vi "DidMotorCompleteWithoutError.vi"(8 "error in (no error)":errorcluster, 11 "MotorController in":refnum<class "MotorController.lvclass">) -> (0 "error out":errorcluster, 2 "Completed Sucessfully":bool, 3 "MotorController out":refnum<class "MotorController.lvclass">)   [LabVIEW 2019, in "MotorController.lvclass"]
uses:
  MotorController.lvclass
  MotorController.lvclass/MotorController.ctl
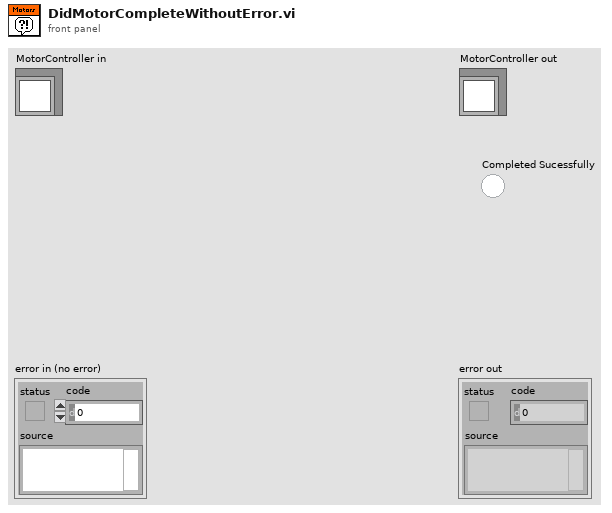
[diagram p1: front panel]
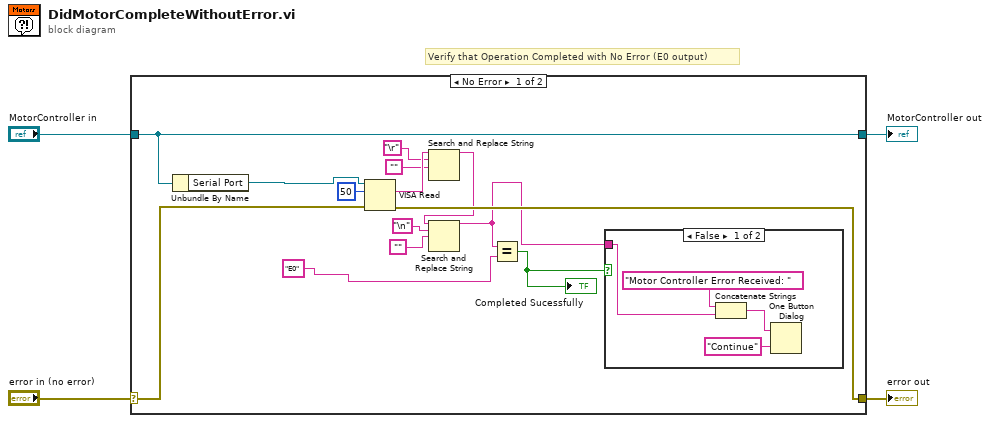
[diagram p0: block diagram]
diagram:
  # "Verify that Operation Completed with No Error (E0 output)"
  n1 = case shown="No Error" "error in (no error)" {
    selector: "error in (no error)" -> [w5 w24]
    tunnel: [w15 w24] -> w3
    tunnel: [w18 w23] -> w1
    tunnel: "MotorController in" -> [w18 w23]
    frame No Error {
      n2 = Unbundle By Name(w18) -> ("Serial Port"=w6:refnum<visa-resource-name>)
      n3 = VISA Read(VISA resource name=w6, byte count=u32 50, error in (no error)=w5) -> (read buffer=w14:string, error out=w15:errorcluster)  [unwired: 2 out]
      n4 = Search and Replace String(input string=w14, search string="\r", replace string="") -> (result string=w10:string)  [unwired: 5 in, 3 out]
      n5 = Search and Replace String(input string=w10, search string="\n", replace string="") -> (result string=w7:string)  [unwired: 5 in, 3 out]
      n6 = Equal?(x=w7, y="E0") -> (x = y?=w17:bool)
      "Completed Sucessfully" <- w17
      n7 = case shown="False" w17 {
        tunnel: w7 -> [w19 _]
        frame False {
          n8 = Concatenate Strings("Motor Controller Error Received: ", w19) -> (w21:string)
          n9 = One Button Dialog(message=w21, button name ("OK")="Continue") -> ()  [unwired: 1 out]
        }
        frame True {
        }
      }
    }
    frame Error {
    }
  }
  "error out" <- w3
  "MotorController out" <- w1
